vi "Actuator-Main.vi"(8 "error in":errorcluster) -> (0 "error out":errorcluster)   [LabVIEW 2021]
doc: "Use this template to build a simple state machine design pattern. Each state executes code and determines which state to transition to."
uses:
  Controls/Actuator-State.ctl
  Controls/Actuator-Data.ctl
  Actuator Module.lvlib
panel:
  out "Status":string
  out "Actuator Display":dbl
  in  "Actuator %":dbl(slide) scale=0.0..100.0
  in  "Exit":bool
  # "Percentage"
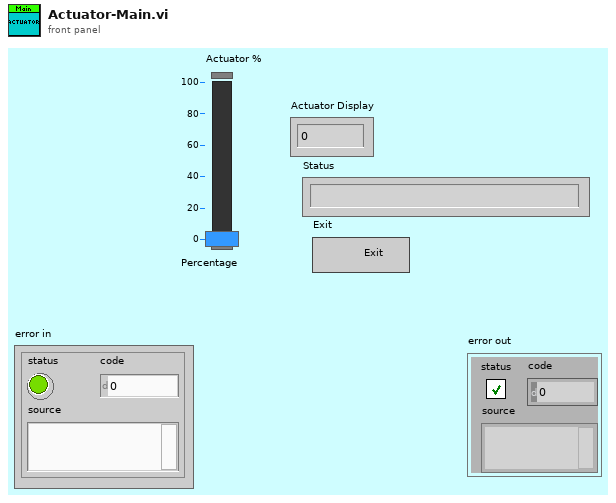
[diagram p1: front panel]
types:
  T1 = typedef "Actuator-Data.ctl" = cluster{"?":bool, "Status":string, "Actuator":dbl}
  T2 = typedef "Actuator-State.ctl" = enum16{"Initialize RS232", "Wait for Event", "Actuator", "Close RS232", "Exit"}
  T3 = typedef "Actuator Module.lvlib/Request Events--cluster.ctl" = cluster{"Stop":refnum<user-event>, "Set Actuator":refnum<user-event>}
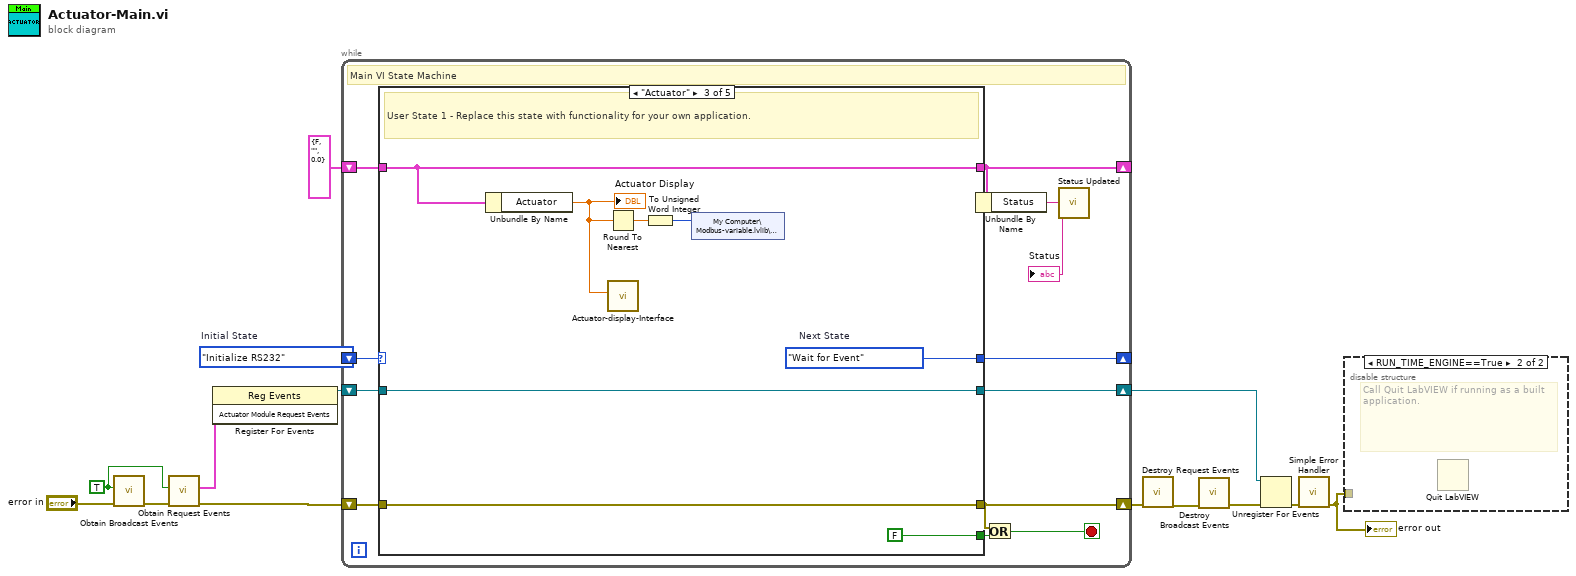
[diagram p0: block diagram]
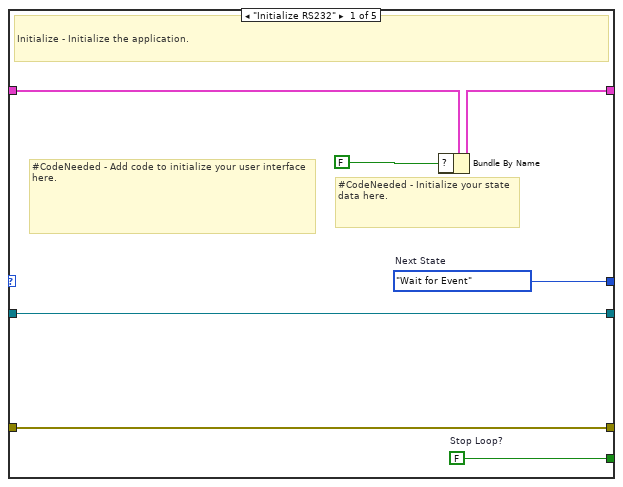
[diagram p3: hidden frame]
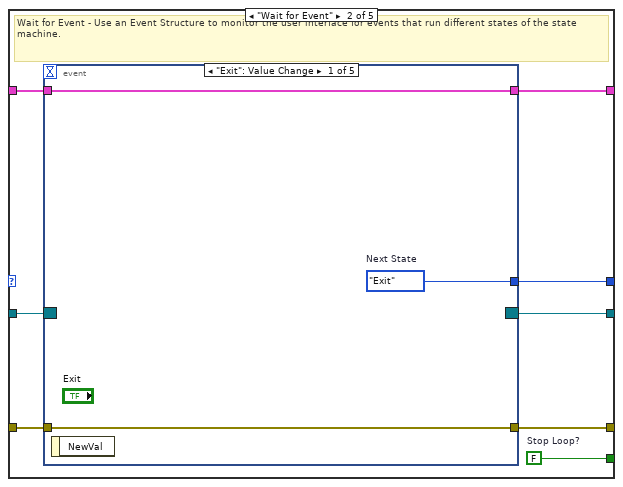
[diagram p4: hidden frame]
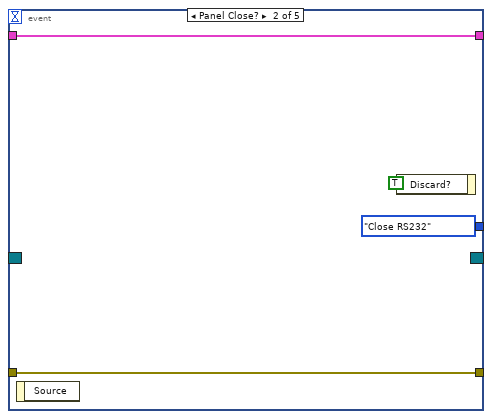
[diagram p5: hidden frame]
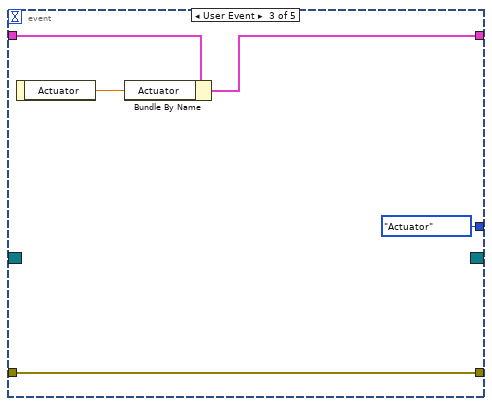
[diagram p6: hidden frame]
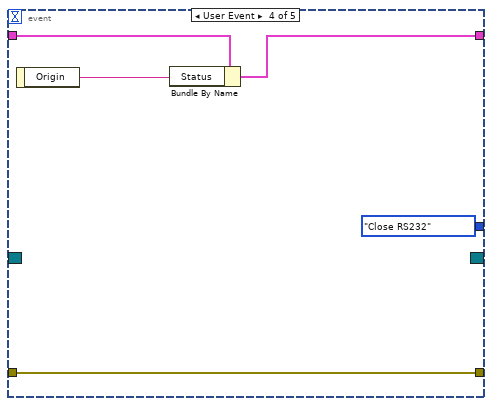
[diagram p7: hidden frame]
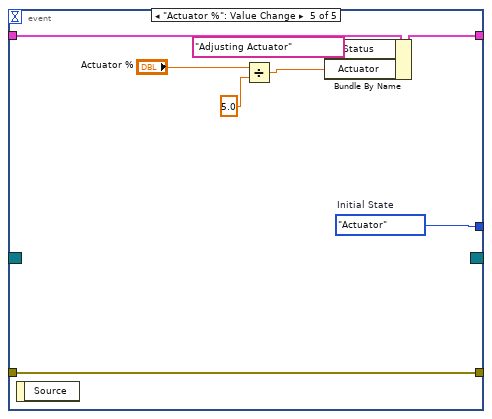
[diagram p8: hidden frame]
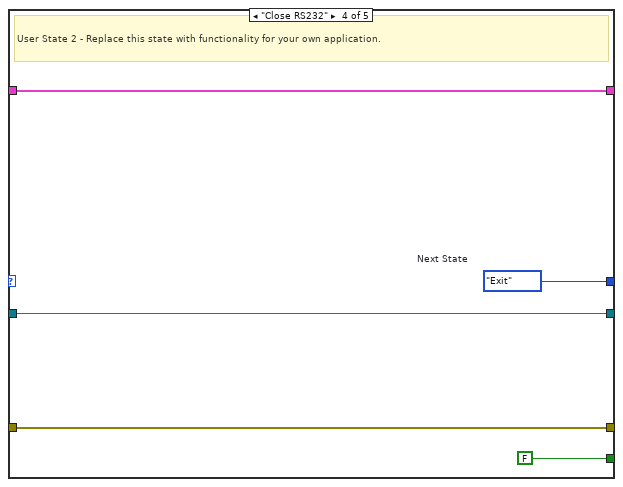
[diagram p9: hidden frame]
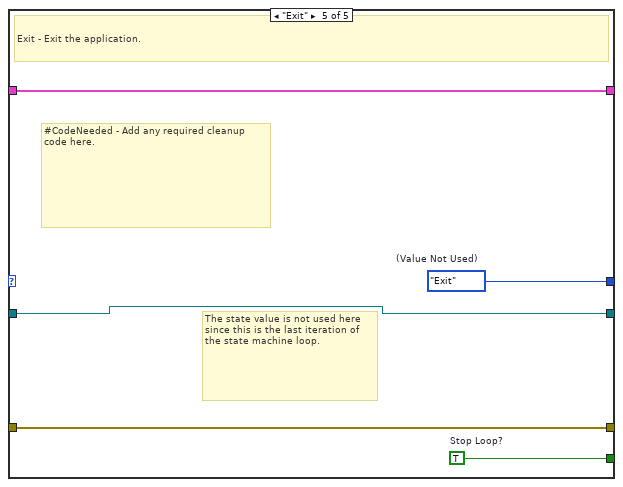
[diagram p10: hidden frame]
diagram:
  w6 = TRUE ("Create New?")
  w14 = Actuator-State."Initialize RS232"  # Initial State
  n1 = call "Obtain Broadcast Events.vi"("error in (no error)"="error in", "Create New?"=w6) -> ("error out"=w10:errorcluster)  [unwired: 8 in, 1 out]
  n2 = call "Obtain Request Events.vi"("error in (no error)"=w10, "Create New?"=w6) -> ("error out"=w8:errorcluster, "Actuator Module Request Events"=w7:T3)  [unwired: 8 in]
  n3 = register-events(w7) -> (reference out=w11:refnum<event-registration>)  [unwired: 2 in, 1 out]
  n4 = while {
    shift-right: [w24] -> _
    shift-left: w14 -> [w25]
    shift-right: [w17] -> _
    shift-left: T1 {"?"=FALSE, "Status"="", "Actuator"=0.0} ("Data") -> [w23]
    shift-right: [w19] -> w3
    shift-left: w8 -> [w22]
    shift-right: [w15] -> w1
    shift-left: w11 -> [w18]
    stop <- w20 stop-if-true
    # "Main VI State Machine"
    n5 = case shown="\"Actuator\"" w25 {
      tunnel: [w32 w40 w73 w78 w83] -> w24
      tunnel: [w31 w39 FALSE ("Stop Loop?") FALSE ("Stop Loop?") w81] -> w21
      tunnel: w23 -> [w30 w38 w71 w76 w82]
      tunnel: [w29 w37 w71 w76 w82] -> w17
      tunnel: w22 -> [w27 w36 w70 w75 w80]
      tunnel: [w27 w35 w70 w75 w80] -> w19
      tunnel: w18 -> [w26 w34 w69 w74 w79]
      tunnel: [w26 w33 w69 w74 w79] -> w15
      frame "Initialize RS232" {
        w31 = FALSE  # Stop Loop?
        w32 = Actuator-State."Wait for Event"  # Next State
        # "#CodeNeeded - Initialize your state data here."
        # "#CodeNeeded - Add code to initialize your user interface here."
        # "Initialize - Initialize the application."
        n6 = Bundle By Name(cluster=w30, "?"=FALSE ("Replace_Me_Boolean")) -> (w29:T1)
      }
      frame "Wait for Event" {
        w39 = FALSE  # Stop Loop?
        # "Wait for Event - Use an Event Structure to monitor the user interface for events that run different states of the state machine."
        n7 = event shown="[0] \"Exit\": Value Change" {
          selector: w34 -> [_ _ _ _ _]
          dyn-events: [_ _ _ _ _] -> w33
          timeout: _ -> [_ _ _ _ _]
          tunnel: [w43 Actuator-State."Close RS232" ("Initial State") Actuator-State."Actuator" ("Initial State") Actuator-State."Close RS232" ("Initial State") w61] -> w40
          tunnel: w38 -> [w42 w47 w51 w56 w65]
          tunnel: [w42 w47 w50 w55 w64] -> w37
          tunnel: w36 -> [w41 w46 w52 w57 w62]
          tunnel: [w41 w46 w52 w57 w62] -> w35
          event "Exit": Value Change {
            w43 = Actuator-State."Exit"  # Next State
            n8 = event-data() -> ()  [unwired: 1 in, 1 out]
          }
          event Panel Close? {
            n9 = event-data() -> ()  [unwired: 1 in, 1 out]
            n10 = event-data("Discard?"=TRUE) -> ()  [unwired: 1 in, 1 out]
          }
          event User Event {
            n11 = event-data() -> ("Actuator"=w49:dbl)  [unwired: 1 in]
            n12 = Bundle By Name(cluster=w51, "Actuator"=w49) -> (w50:T1)
          }
          event User Event {
            n13 = event-data() -> ("Origin"=w54:string)  [unwired: 1 in]
            n14 = Bundle By Name(cluster=w56, "Status"=w54) -> (w55:T1)
          }
          event "Actuator %": Value Change {
            w61 = Actuator-State."Actuator"  # Initial State
            n15 = event-data() -> ()  [unwired: 1 in, 1 out]
            n16 = Divide(x="Actuator %", y=5.0) -> (x/y=w59:dbl)
            n17 = Bundle By Name(cluster=w65, "Status"="Adjusting Actuator" ("Running User State 1"), "Actuator"=w59) -> (w64:T1)
          }
        }
      }
      frame "Actuator" {
        w73 = Actuator-State."Wait for Event"  # Next State
        # "User State 1 - Replace this state with functionality for your own application."
        n18 = Unbundle By Name(w71) -> ("Actuator"=w68:dbl)
        "Actuator Display" <- w68
        n19 = Round To Nearest(number=w68) -> (nearest integer value=w66:dbl)
        n20 = call "Actuator-display-Interface.vi"("Actuator"=w68) -> ()  [unwired: 10 in, 1 out]
        n21 = To Unsigned Word Integer(number=w66) -> (unsigned 16bit integer=w67:u16)
        n22 = shared-variable "My Computer\\Modbus-variable.lvlib\\400009"(w67) -> ()  [unwired: 1 in, 1 out]
      }
      frame "Close RS232" {
        w78 = Actuator-State."Exit"  # Next State
        # "User State 2 - Replace this state with functionality for your own application."
      }
      frame "Exit" {
        w81 = TRUE  # Stop Loop?
        w83 = Actuator-State."Exit"  # (Value Not Used)
        # "#CodeNeeded - Add any required cleanup code here."
        # "The state value is not used here since this is the last iteration of the state machine loop."
        # "Exit - Exit the application."
      }
    }
    n23 = Unbundle By Name(w17) -> ("Status"=w16:string)
    "Status" <- w16
    n24 = Or(x=w19, y=w21) -> (x .or. y?=w20:bool)
    n25 = call "Status Updated.vi"("Status"=w16) -> ()  [unwired: 10 in, 1 out]
  }
  n26 = call "Destroy Request Events.vi"("error in (no error)"=w3) -> ("error out"=w5:errorcluster)  [unwired: 10 in]
  n27 = call "Destroy Broadcast Events.vi"("error in (no error)"=w5) -> ("error out"=w4:errorcluster)  [unwired: 10 in]
  n28 = Unregister For Events(event registration refnum=w1, error in=w4) -> (error out=w2:errorcluster)
  n29 = call <vilib>:"Simple Error Handler.vi"("error in (no error)"=w2) -> ("error out"=w12:errorcluster)  [unwired: 4 in, 4 out]
  "error out" <- w12
  n30 = disable-structure shown="RUN_TIME_ENGINE==True" {
    disable-tunnel: w12 -> [_ _]
    frame condition #0 (active) {
    }
    frame condition #1 {
      # "Call Quit LabVIEW if running as a built application."
      n31 = Quit LabVIEW() -> ()  [unwired: 1 in]
    }
  }
